vi "GEOM_SingleFPA2DetROI.vi"(9 "FPAROIcoords":T2, 10 "FPAampcoords":cluster{"Xs":i32, "Ys":i32, "Xe":i32, "Ye":i32}) -> (1 "ROI det size":cluster{"xrs":i32, "yrs":i32, i32, i32}, 2 "ROI det coords":T1)   [LabVIEW 2016]
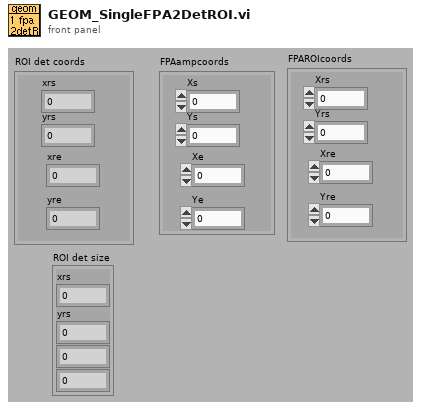
[diagram p1: front panel]
types:
  T1 = cluster{"xrs":i32, "yrs":i32, "xre":i32, "yre":i32}
  T2 = cluster{"Xrs":i32, "Yrs":i32, "Xre":i32, "Yre":i32}
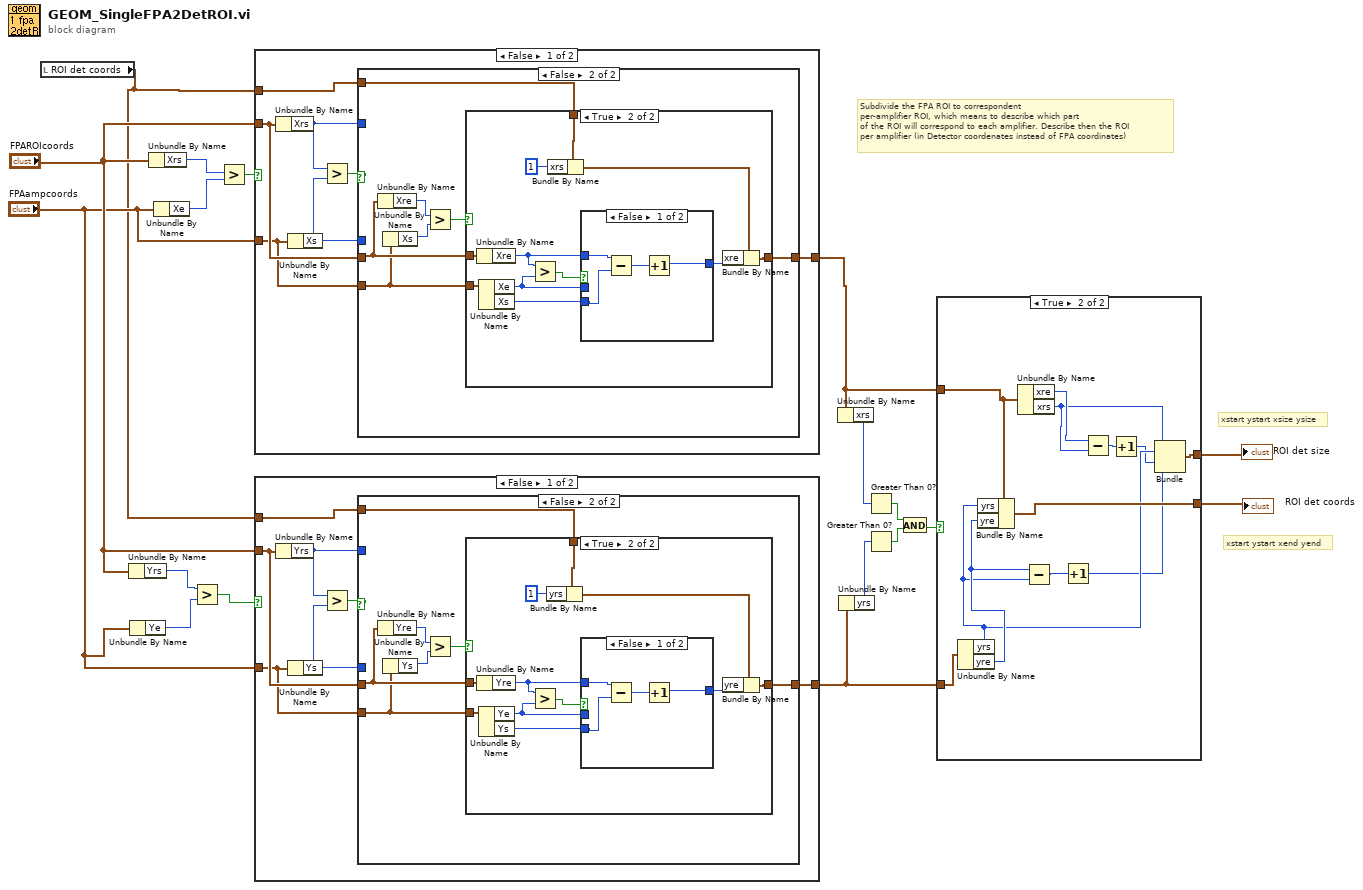
[diagram p0: block diagram]
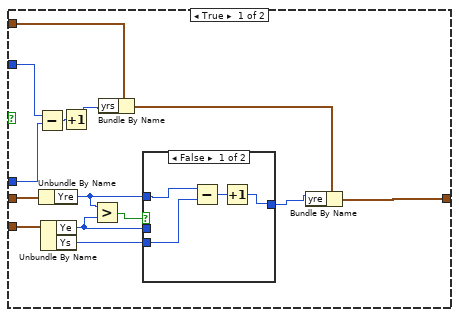
[diagram p2: hidden frame]
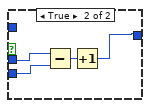
[diagram p3: hidden frame]
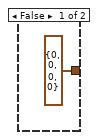
[diagram p4: hidden frame]
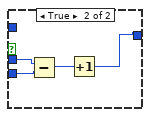
[diagram p5: hidden frame]
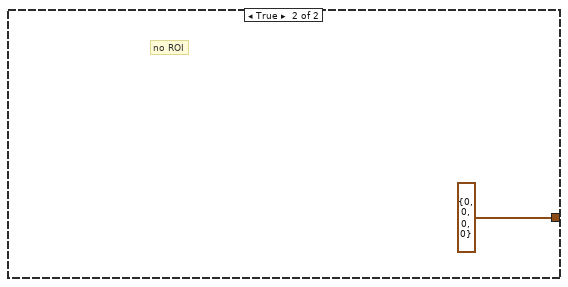
[diagram p6: hidden frame]
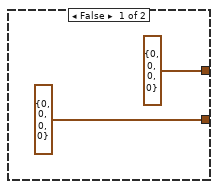
[diagram p7: hidden frame]
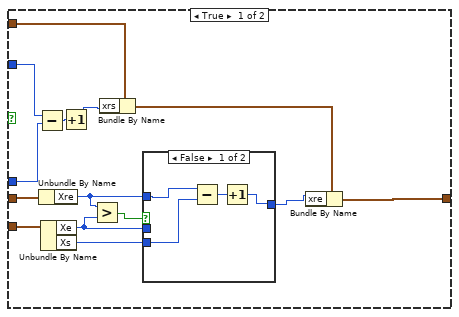
[diagram p8: hidden frame]
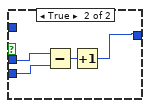
[diagram p9: hidden frame]
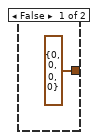
[diagram p10: hidden frame]
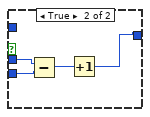
[diagram p11: hidden frame]
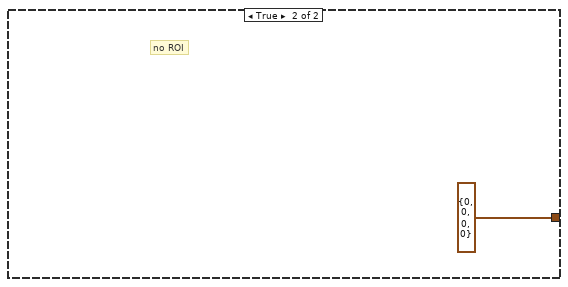
[diagram p12: hidden frame]
diagram:
  # "Subdivide the FPA ROI to correspondent\nper-amplifier ROI, which means to describe which part\nof the ROI will correspond to each amplifier. Describe then the ROI\nper amplifier (in Detector coordenates instead of FPA coordinates)"
  # "xstart ystart xend yend"
  # "xstart ystart xsize ysize"
  n1 = local read "ROI det coords"() -> (w3:T1)
  n2 = Unbundle By Name("FPAROIcoords") -> ("Yrs"=w15:i32)
  n3 = Unbundle By Name("FPAampcoords") -> ("Ye"=w14:i32)
  n4 = Unbundle By Name("FPAROIcoords") -> ("Xrs"=w18:i32)
  n5 = Unbundle By Name("FPAampcoords") -> ("Xe"=w17:i32)
  n6 = Greater?(x=w15, y=w14) -> (0:w8:bool)
  n7 = Greater?(x=w18, y=w17) -> (0:w16:bool)
  n8 = case shown="False" w16 {
    tunnel: "FPAROIcoords" -> [w21 _]
    tunnel: "FPAampcoords" -> [w20 _]
    tunnel: w3 -> [w22 _]
    tunnel: [w19 T1 {"xrs"=0, "yrs"=0, "xre"=0, "yre"=0} ("DETampcoords")] -> w9
    frame False {
      n9 = Unbundle By Name(w21) -> ("Xrs"=w25:i32)
      n10 = Unbundle By Name(w20) -> ("Xs"=w24:i32)
      n11 = Greater?(x=w25, y=w24) -> (0:w23:bool)
      n12 = case shown="False" w23 {
        tunnel: w22 -> [w39 w54]
        tunnel: w25 -> [w38 _]
        tunnel: w24 -> [w37 _]
        tunnel: w21 -> [w34 w52]
        tunnel: w20 -> [w33 w51]
        tunnel: [w26 w53] -> w19
        frame True {
          n13 = Subtract(x=w38, y=w37) -> (x-y=w36:i32)
          n14 = Unbundle By Name(w34) -> ("Xre"=w31:i32)
          n15 = Unbundle By Name(w33) -> ("Xe"=w30:i32, "Xs"=w27:i32)
          n16 = Increment(x=w36) -> (x+1=w35:i32)
          n17 = Greater?(x=w31, y=w30) -> (0:w32:bool)
          n18 = Bundle By Name(cluster=w39, "xrs"=w35) -> (w29:T1)
          n19 = case shown="False" w32 {
            tunnel: w31 -> [w41 _]
            tunnel: w30 -> [_ w47]
            tunnel: [w42 w44] -> w28
            tunnel: w27 -> [w40 w46]
            frame False {
              n20 = Subtract(x=w41, y=w40) -> (x-y=w43:i32)
              n21 = Increment(x=w43) -> (x+1=w42:i32)
            }
            frame True {
              n22 = Subtract(x=w47, y=w46) -> (x-y=w45:i32)
              n23 = Increment(x=w45) -> (x+1=w44:i32)
            }
          }
          n24 = Bundle By Name(cluster=w29, "xre"=w28) -> (w26:T1)
        }
        frame False {
          n25 = Unbundle By Name(w52) -> ("Xre"=w49:i32)
          n26 = Unbundle By Name(w51) -> ("Xs"=w48:i32)
          n27 = Greater?(x=w49, y=w48) -> (0:w50:bool)
          n28 = case shown="True" w50 {
            tunnel: w54 -> [_ w66]
            tunnel: w52 -> [_ w65]
            tunnel: w51 -> [_ w64]
            tunnel: [T1 {"xrs"=0, "yrs"=0, "xre"=0, "yre"=0} ("DETampcoords") w56] -> w53
            frame False {
            }
            frame True {
              n29 = Unbundle By Name(w65) -> ("Xre"=w62:i32)
              n30 = Unbundle By Name(w64) -> ("Xe"=w61:i32, "Xs"=w57:i32)
              n31 = Greater?(x=w62, y=w61) -> (0:w63:bool)
              n32 = Bundle By Name(cluster=w66, "xrs"=1) -> (w60:T1)
              n33 = case shown="False" w63 {
                tunnel: w62 -> [w70 _]
                tunnel: w61 -> [_ w74]
                tunnel: [w68 w71] -> w59
                tunnel: w57 -> [w67 w73]
                frame False {
                  n34 = Subtract(x=w70, y=w67) -> (x-y=w69:i32)
                  n35 = Increment(x=w69) -> (x+1=w68:i32)
                }
                frame True {
                  n36 = Subtract(x=w74, y=w73) -> (x-y=w72:i32)
                  n37 = Increment(x=w72) -> (x+1=w71:i32)
                }
              }
              n38 = Bundle By Name(cluster=w60, "xre"=w59) -> (w56:T1)
            }
          }
        }
      }
    }
    frame True {
      # "no ROI"
    }
  }
  n39 = case shown="False" w8 {
    tunnel: "FPAROIcoords" -> [w78 _]
    tunnel: "FPAampcoords" -> [w77 _]
    tunnel: w3 -> [w79 _]
    tunnel: [w76 T1 {"xrs"=0, "yrs"=0, "xre"=0, "yre"=0} ("DETampcoords")] -> w4
    frame False {
      n40 = Unbundle By Name(w78) -> ("Yrs"=w82:i32)
      n41 = Unbundle By Name(w77) -> ("Ys"=w81:i32)
      n42 = Greater?(x=w82, y=w81) -> (0:w80:bool)
      n43 = case shown="False" w80 {
        tunnel: w79 -> [w96 w111]
        tunnel: w82 -> [w95 _]
        tunnel: w81 -> [w94 _]
        tunnel: w78 -> [w91 w109]
        tunnel: w77 -> [w90 w108]
        tunnel: [w83 w110] -> w76
        frame True {
          n44 = Subtract(x=w95, y=w94) -> (x-y=w93:i32)
          n45 = Unbundle By Name(w91) -> ("Yre"=w88:i32)
          n46 = Unbundle By Name(w90) -> ("Ye"=w87:i32, "Ys"=w84:i32)
          n47 = Increment(x=w93) -> (x+1=w92:i32)
          n48 = Greater?(x=w88, y=w87) -> (0:w89:bool)
          n49 = Bundle By Name(cluster=w96, "yrs"=w92) -> (w86:T1)
          n50 = case shown="False" w89 {
            tunnel: w88 -> [w98 _]
            tunnel: w87 -> [_ w104]
            tunnel: [w99 w101] -> w85
            tunnel: w84 -> [w97 w103]
            frame False {
              n51 = Subtract(x=w98, y=w97) -> (x-y=w100:i32)
              n52 = Increment(x=w100) -> (x+1=w99:i32)
            }
            frame True {
              n53 = Subtract(x=w104, y=w103) -> (x-y=w102:i32)
              n54 = Increment(x=w102) -> (x+1=w101:i32)
            }
          }
          n55 = Bundle By Name(cluster=w86, "yre"=w85) -> (w83:T1)
        }
        frame False {
          n56 = Unbundle By Name(w109) -> ("Yre"=w106:i32)
          n57 = Unbundle By Name(w108) -> ("Ys"=w105:i32)
          n58 = Greater?(x=w106, y=w105) -> (0:w107:bool)
          n59 = case shown="True" w107 {
            tunnel: w111 -> [_ w123]
            tunnel: w109 -> [_ w122]
            tunnel: w108 -> [_ w121]
            tunnel: [T1 {"xrs"=0, "yrs"=0, "xre"=0, "yre"=0} ("DETampcoords") w113] -> w110
            frame False {
            }
            frame True {
              n60 = Unbundle By Name(w122) -> ("Yre"=w119:i32)
              n61 = Unbundle By Name(w121) -> ("Ye"=w118:i32, "Ys"=w114:i32)
              n62 = Greater?(x=w119, y=w118) -> (0:w120:bool)
              n63 = Bundle By Name(cluster=w123, "yrs"=1 ("xrs")) -> (w117:T1)
              n64 = case shown="False" w120 {
                tunnel: w119 -> [w127 _]
                tunnel: w118 -> [_ w131]
                tunnel: [w125 w128] -> w116
                tunnel: w114 -> [w124 w130]
                frame False {
                  n65 = Subtract(x=w127, y=w124) -> (x-y=w126:i32)
                  n66 = Increment(x=w126) -> (x+1=w125:i32)
                }
                frame True {
                  n67 = Subtract(x=w131, y=w130) -> (x-y=w129:i32)
                  n68 = Increment(x=w129) -> (x+1=w128:i32)
                }
              }
              n69 = Bundle By Name(cluster=w117, "yre"=w116) -> (w113:T1)
            }
          }
        }
      }
    }
    frame True {
      # "no ROI"
    }
  }
  n70 = Unbundle By Name(w9) -> ("xrs"=w13:i32)
  n71 = Unbundle By Name(w4) -> ("yrs"=w5:i32)
  n72 = Greater Than 0?(x=w13) -> (x > 0?=w11:bool)
  n73 = Greater Than 0?(x=w5) -> (x > 0?=w10:bool)
  n74 = And(x=w11, y=w10) -> (x .and. y?=w12:bool)
  n75 = case shown="True" w12 {
    tunnel: w9 -> [_ w141]
    tunnel: [T1 {"xrs"=0, "yrs"=0, "xre"=0, "yre"=0} ("DETampcoords") w146] -> w1
    tunnel: w4 -> [_ w145]
    tunnel: [cluster{"xrs":i32, "yrs":i32, i32, i32} {"xrs"=0, "yrs"=0, 0, 0} w135] -> w2
    frame False {
    }
    frame True {
      n76 = Unbundle By Name(w145) -> ("yrs"=w138:i32, "yre"=w143:i32)
      n77 = Bundle By Name(cluster=w141, "yrs"=w138, "yre"=w143) -> (w146:T1)
      n78 = Unbundle By Name(w141) -> ("xre"=w140:i32, "xrs"=w139:i32)
      n79 = Subtract(x=w143, y=w138) -> (x-y=w144:i32)
      n80 = Increment(x=w144) -> (x+1=w136:i32)
      n81 = Subtract(x=w140, y=w139) -> (x-y=w142:i32)
      n82 = Increment(x=w142) -> (x+1=w137:i32)
      n83 = Bundle("xrs"=w139, "yrs"=w138, w137, w136) -> (w135:cluster{"xrs":i32, "yrs":i32, i32, i32})  [unwired: 1 out]
    }
  }
  "ROI det coords" <- w1
  "ROI det size" <- w2
